vi "Set AO Sampling Rate.vi"(8 "error in (no error)":errorcluster, 10 "Fs (Hz)":dbl, 11 "State in":refnum<class "State.lvclass">) -> (0 "error out":errorcluster, 3 "State out":refnum<class "State.lvclass">)   [LabVIEW 2020, in "State.lvclass"]
uses:
  State.lvclass
  State.lvclass/State.ctl
  epl-vi-lib/Signal Synthesis VIs/4th Generation/Classes/SignalManager/SignalManager.lvclass/SignalManager.ctl
  epl-vi-lib/Signal Synthesis VIs/4th Generation/Classes/SignalManager/Write Fs (Hz).vi
  epl-vi-lib/Signal Synthesis VIs/4th Generation/Classes/SignalManager/SignalManager.lvclass
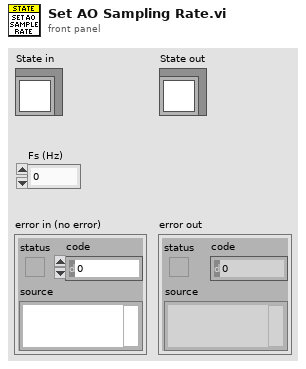
[diagram p1: front panel]
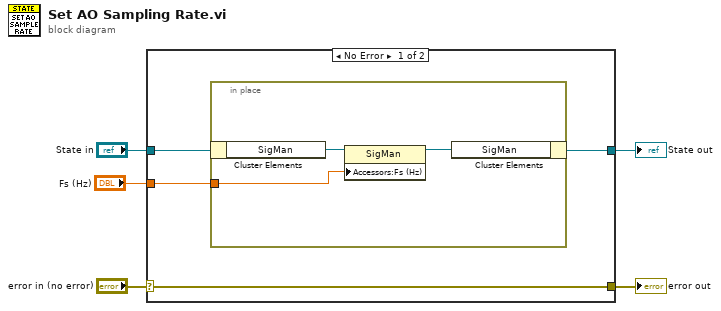
[diagram p0: block diagram]
diagram:
  n1 = case shown="No Error" "error in (no error)" {
    selector: "error in (no error)" -> [w9 w14]
    tunnel: [w9 w14] -> w4
    tunnel: [w7 w13] -> w2
    tunnel: "State in" -> [w8 w13]
    tunnel: "Fs (Hz)" -> [w6 _]
    frame No Error {
      n2 = in-place {
        in-place-border: w6 -> [w10]
        n3 = in-place-cluster #1(w8) -> ("SigMan"=w12:refnum<class "SignalManager.lvclass">)
        n4 = property class="SigMan"(reference=w12, "Accessors:Fs (Hz)"=w10) -> (reference out=w11:refnum<class "SignalManager.lvclass">)  [unwired: 1 in, 1 out]
        n5 = in-place-cluster #1("SigMan"=w11) -> (w7:refnum<class "State.lvclass">)
      }
    }
    frame Error {
    }
  }
  "error out" <- w4
  "State out" <- w2
